vi "Example G-CLI.vi"() -> ()   [LabVIEW 2013]
uses:
  <vilib>/Utility/sysdir.llb/System Directory Type.ctl
panel:
  out "return code":i32
  out "standard output":string
  in  "LabVIEW Version":u16=2019
  out "Command Line string":string
  in  "Output file":path
  out "error out":errorcluster
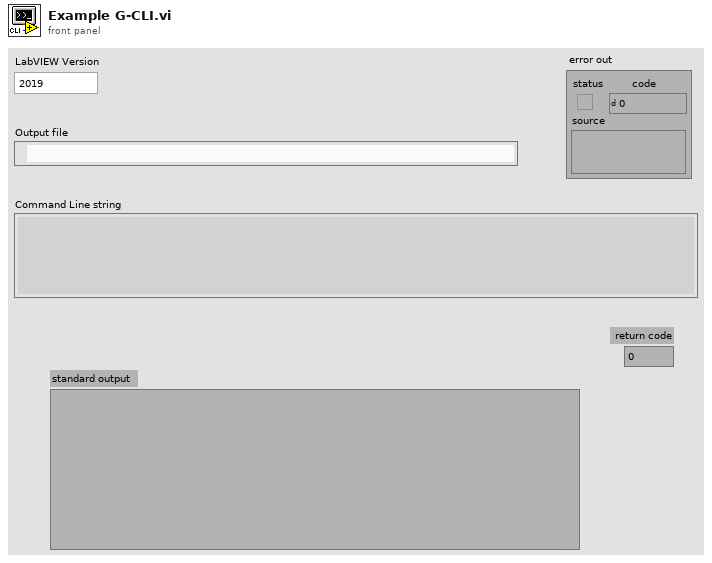
[diagram p1: front panel]
types:
  T1 = typedef "System Directory Type.ctl" = i32
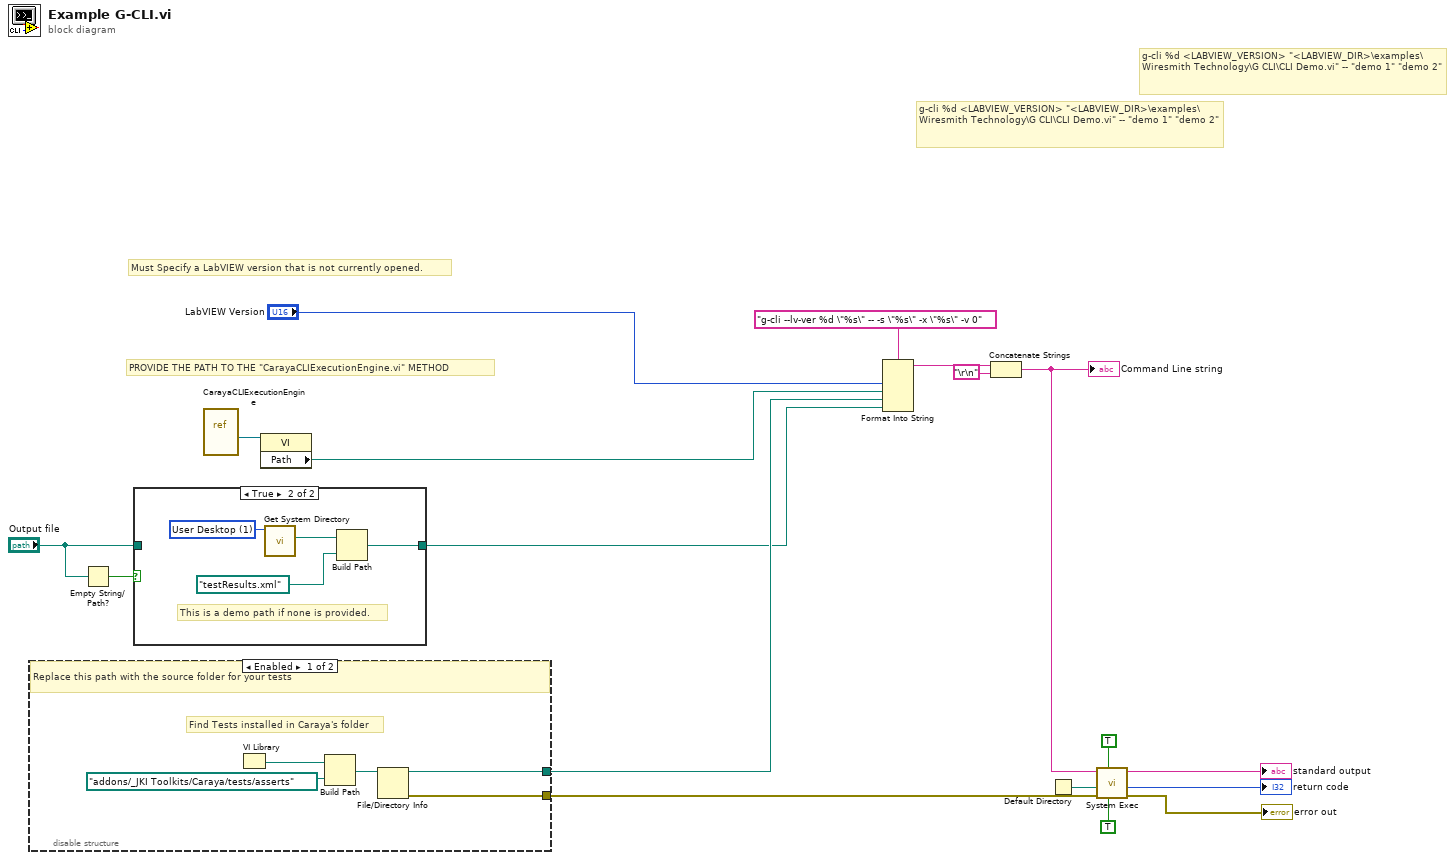
[diagram p0: block diagram]
diagram:
  # "PROVIDE THE PATH TO THE \"CarayaCLIExecutionEngine.vi\" METHOD"
  # "g-cli %d <LABVIEW_VERSION> \"<LABVIEW_DIR>\\examples\\Wiresmith Technology\\G CLI\\CLI Demo.vi\" -- \"demo 1\" \"demo 2\""
  # "g-cli %d <LABVIEW_VERSION> \"<LABVIEW_DIR>\\examples\\Wiresmith Technology\\G CLI\\CLI Demo.vi\" -- \"demo 1\" \"demo 2\""
  # "Must Specify a LabVIEW version that is not currently opened."
  n1 = disable-structure shown="Enabled" {
    disable-tunnel: [w23 _] -> w6
    disable-tunnel: [w19 _] -> w2
    frame Enabled {
      # "Find Tests installed in Caraya's folder"
      # "Replace this path with the source folder for your tests"
      n2 = VI Library() -> (path=w22:path)
      n3 = Build Path(base path=w22, name or relative path=path "addons/_JKI Toolkits/Caraya/tests/asserts") -> (appended path=w20:path)
      n4 = File/Directory Info(path=w20) -> (path out=w23:path, error out=w19:errorcluster)  [unwired: 1 in, 5 out]
    }
    frame Disabled {
    }
  }
  n5 = Empty String/Path?(string/path="Output file") -> (empty?=w9:bool)
  n6 = case shown="True" w9 {
    tunnel: [w24 w26] -> w3
    tunnel: "Output file" -> [w24 _]
    frame False {
    }
    frame True {
      w28 = T1 1 items=["User Home"=0, "User Desktop"=1, "User Documents"=2, "User Application Data"=3, "User Preferences"=4, "User Temporary"=5, "Public Documents"=6, "Public Application Data"=7, "Public Preferences"=8, "Public Cache"=13, "System Core Libraries"=9, "System Installed Libraries"=10, "Application Files"=11, "Boot Volume Root"=12] ("system directory type")
      # "This is a demo path if none is provided."
      n7 = call <vilib>:"Get System Directory.vi"("system directory type"=w28) -> ("system directory"=w25:path)  [unwired: 10 in]
      n8 = Build Path(base path=w25, name or relative path=path "testResults.xml") -> (appended path=w26:path)
    }
  }
  n9 = vi-ref "CarayaCLIExecutionEngine.vi"() -> (w1:refnum<vi>)
  n10 = property class="VI"(reference=w1) -> ("Path"=w10:path)  [unwired: 1 in, 2 out]
  n11 = Format Into String(format string="g-cli --lv-ver %d \"%s\" -- -s \"%s\" -x \"%s\" -v 0", "LabVIEW Version", w10, w6, w3) -> (resulting string=w12:string)  [unwired: 2 in, 1 out]
  n12 = Concatenate Strings(w12, "\r\n") -> (w14:string)
  "Command Line string" <- w14
  n13 = Default Directory() -> (w11:path)
  n14 = call <vilib>:"System Exec.vi"("run minimized? (F)"=TRUE, "wait until completion? (T)"=TRUE, "error in (no error)"=w2, "working directory"=w11, "command line"=w14) -> ("error out"=→"error out":errorcluster, "return code"=→"return code":i32, "standard output"=→"standard output":string)  [unwired: 3 in, 1 out]
